vi "GetText.vi"(8 "error in":errorcluster, 11 "Temperature in":refnum<class "Temperature.lvclass">) -> (0 "error out":errorcluster, 1 "additional text":string, 2 "text":string, 3 "Temperature out":refnum<class "Temperature.lvclass">, 4 "glyph":string)   [LabVIEW 2015, in "Temperature.lvclass"]
uses:
  Temperature.lvclass
  Channel/Channel.lvclass
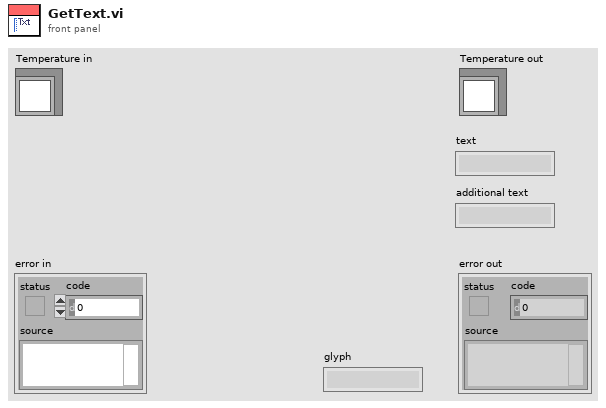
[diagram p1: front panel]
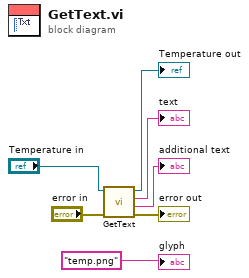
[diagram p0: block diagram]
diagram:
  n1 = call-parent "GetText.vi"("error in"="error in", "channel in"="Temperature in") -> ("error out"=→"error out":errorcluster, "additional text"=→"additional text":string, "text"=→"text":string, "channel out"=→"Temperature out":refnum<class "Temperature.lvclass">)  [unwired: 5 in, 1 out]
  "glyph" <- "temp.png" ("glyph")
